vi "Copy (No Check).vi"(8 "error in (no error)":errorcluster, 9 "bytes to copy":u64 format="%08x bytes", 10 "dst Pointer in":refnum<class "Pointer.lvclass">, 11 "src Pointer in":refnum<class "Pointer.lvclass">) -> (0 "error out":errorcluster, 1 "bytes to copy":u64 format="%08x bytes", 2 "dst Pointer out":refnum<class "Pointer.lvclass">, 3 "src Pointer out":refnum<class "Pointer.lvclass">)   [LabVIEW 2020, in "Memory Manager.lvlib" / "Pointer.lvclass"]
doc: "Copies <b>bytes to copy</b> of data from the memory address specified by <b>src pointer</b> to the memory address specified by <b>dst pointer</b>.\n\n<b>Note:</b> This VI is <b>unsafe</b>.\n\nUnsafe means that this function does not have a check to ensure that the size of the requested source memory transfer is inbounds of allocated memory for the destination before peforming a memory read/write. Reading/writing more data to a pointer than it has allocated can corrupt or crash LabVIEW. Only use this VI in scenarios where the <b>dst pointer</b> has been validated to be allocated to a correct size before calling this VI."
uses:
  Pointer.lvclass
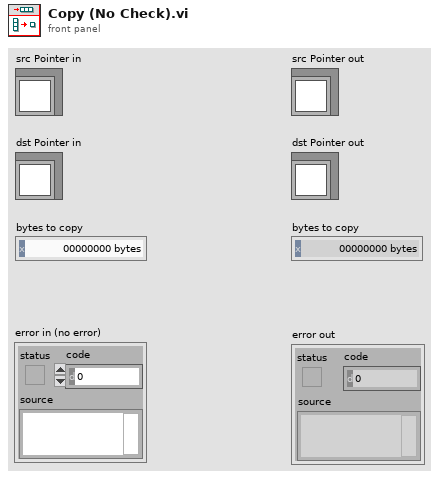
[diagram p1: front panel]
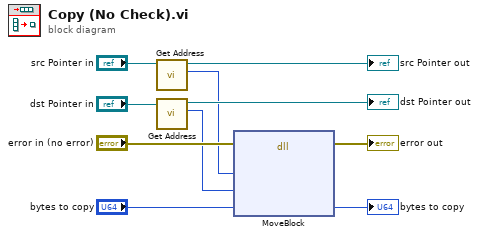
[diagram p0: block diagram]
diagram:
  n1 = call "Get Address.vi"("Pointer in"="src Pointer in") -> ("address"=w3:u64, "Pointer out"=→"src Pointer out":refnum<class "Pointer.lvclass">)  [unwired: 9 in]
  n2 = call "Get Address.vi"("Pointer in"="dst Pointer in") -> ("address"=w4:u64, "Pointer out"=→"dst Pointer out":refnum<class "Pointer.lvclass">)  [unwired: 9 in]
  n3 = dll-call lib="LabVIEW" fn="MoveBlock"(error in="error in (no error)", "src"=w3, "dst"=w4, "size"="bytes to copy") -> (error out=→"error out":errorcluster, "size"=→"bytes to copy":u64)  [unwired: 5 in, 1 out]
